vi "读写信号轮询参数文件.vi"(0 "信号轮询发送设置IN":cluster{"XNET SignalFrameArry":T1[]}={"XNET SignalFrameArry"=[{"Port_No."="CAN1", "计数Count"=TRUE, "校验CheckSum"=TRUE, "MessageFrame"="ESP_1\nLR110", "校验算法名称"="Anti_Add"}, {"Port_No."="CAN1", "计数Count"=FALSE, "校验CheckSum"=FALSE, "MessageFrame"="VTOG_1\nLR110", "校验算法名称"=""}]}, 1 "T:Read/F:Write":bool=TRUE, 5 "error in (no error)":errorcluster caption="错误输入（无错误）") -> (14 "信号轮询发送设置Out":cluster{"XNET SignalFrameArry":T1[]}, 19 "error out":errorcluster caption="错误输出")   [LabVIEW 2020, in "SignalSenderLoop.lvclass"]
uses:
  SignalSenderLoop.lvclass
  subvi/SignalFrameSet.ctl
  <vilib>/Utility/config.llb/NI_LVConfig.lvlib
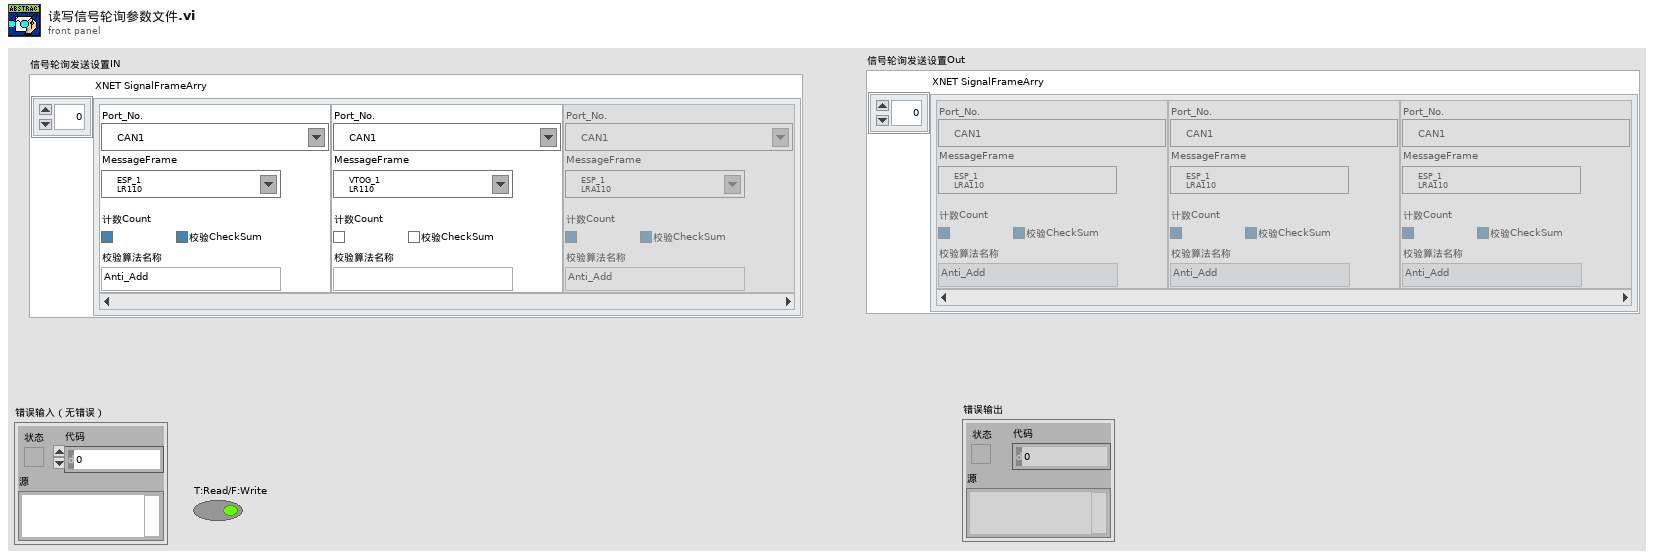
[diagram p1: front panel]
types:
  T1 = typedef "SignalSenderLoop.lvclass/SignalFrameSet.ctl" = cluster{"Port_No.":refnum<k21>, "计数Count":bool, "校验CheckSum":bool, "MessageFrame":refnum<k21>, "校验算法名称":string}
  T2 = enum32{"invalid app kind", "Development System", "Run Time System", "Student Edition", "Embedded LabVIEW", "Evaluation", "Custom"}
  T3 = typedef "NI_LVConfig.lvlib/Config Data RefNum.ctl" = refnum<k1>
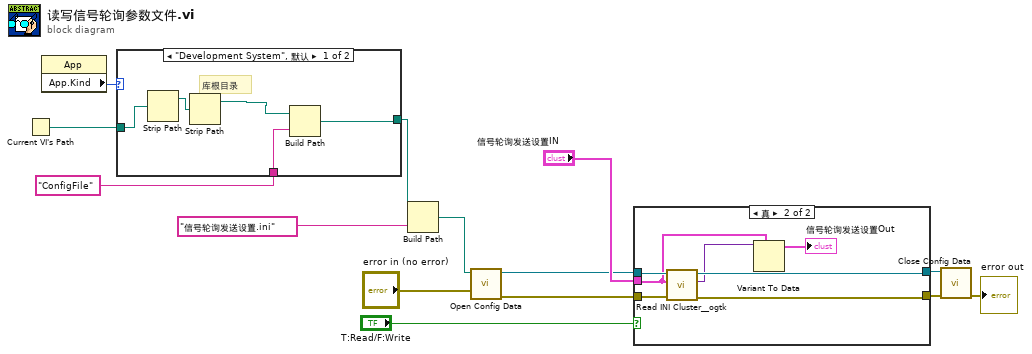
[diagram p0: block diagram]
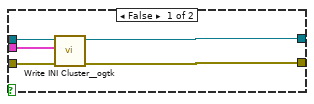
[diagram p2: hidden frame]
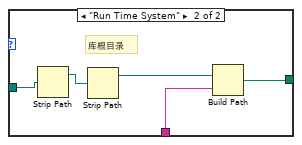
[diagram p3: hidden frame]
diagram:
  n1 = Current VI's Path() -> (path=w8:path)
  n2 = property class="App"() -> ("App.Kind"=w7:T2)  [unwired: 2 in, 2 out]
  n3 = case shown="\"Development System\", 默认" w7 {
    tunnel: w8 -> [w19 w24]
    tunnel: [w16 w20] -> w6
    tunnel: "ConfigFile" ("ConfigFlieFolderName") -> [w15 w21]
    frame "Development System", Default {
      # "库根目录"
      n4 = Strip Path(path=w19) -> (stripped path=w18:path)  [unwired: 1 out]
      n5 = Strip Path(path=w18) -> (stripped path=w17:path)  [unwired: 1 out]
      n6 = Build Path(base path=w17, name or relative path=w15) -> (appended path=w16:path)
    }
    frame "Run Time System" {
      # "库根目录"
      n7 = Strip Path(path=w24) -> (stripped path=w23:path)  [unwired: 1 out]
      n8 = Strip Path(path=w23) -> (stripped path=w22:path)  [unwired: 1 out]
      n9 = Build Path(base path=w22, name or relative path=w21) -> (appended path=w20:path)
    }
  }
  n10 = Build Path(base path=w6, name or relative path="信号轮询发送设置.ini" ("ConfigFlieFolderName")) -> (appended path=w5:path)
  n11 = call <vilib>:"Open Config Data.vi"("error in (no error)"="error in (no error)", "configuration file path"=w5) -> ("error out"=w12:errorcluster, "refnum"=w13:T3)  [unwired: 7 in, 1 out]
  n12 = case shown="真" "T:Read/F:Write" {
    tunnel: "信号轮询发送设置IN" -> [w29 w32]
    tunnel: w13 -> [w28 w36]
    tunnel: w12 -> [w27 w34]
    tunnel: [w26 w35] -> w11
    tunnel: [w25 w33] -> w10
    frame False {
      n13 = call <userlib>:"Write INI Cluster__ogtk.vi"("error in (no error)"=w27, "INI Fomatted Cluster"=w29, "refnum"=w28) -> ("error out"=w25:errorcluster, "dup refnum"=w26:T3)  [unwired: 7 in]
    }
    frame True {
      n14 = call <userlib>:"Read INI Cluster__ogtk.vi"("error in (no error)"=w34, "INI Fomatted Cluster Type"=w32, "refnum"=w36) -> ("error out"=w33:errorcluster, "INI Fomatted Cluster"=w31:variant, "dup refnum"=w35:T3)  [unwired: 4 in, 2 out]
      n15 = Variant To Data(type=w32, Variant=w31) -> (data=→"信号轮询发送设置Out":cluster{"XNET SignalFrameArry":T1[]})  [unwired: 1 in, 1 out]
    }
  }
  n16 = call <vilib>:"Close Config Data.vi"("error in (no error)"=w10, "refnum"=w11) -> ("error out"=→"error out":errorcluster)  [unwired: 8 in, 1 out]
